vi "radio_get.vi"(0 "VISA in":refnum<visa-resource-name>, 2 "Radio get command":u16(ring) items=["op mode", "frequency", "power", "spread factor", "freq correction", "RX signal bw", "bitrate", "freq deviation", "preamble length", "crc", "bandwidth", "snr"], 5 "error in":errorcluster) -> (14 "VISA out":refnum<visa-resource-name>, 16 "response":string="\r\n", 17 "Num out":u32=57600 max=65535 step=1, 18 "Bool out":bool, 19 "error out":errorcluster)   [LabVIEW 2011]
panel:
  out "read buffer":string
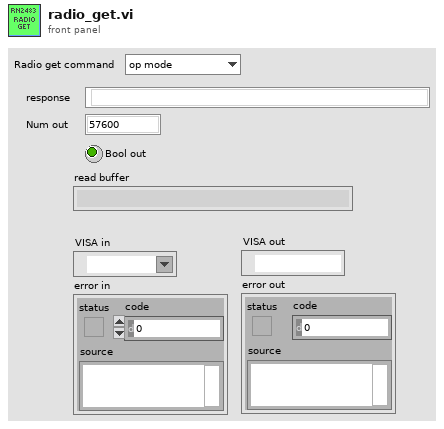
[diagram p1: front panel]
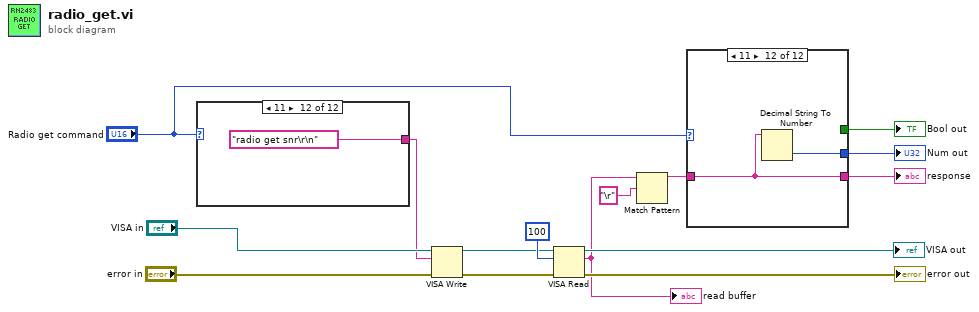
[diagram p0: block diagram]
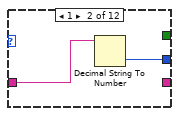
[diagram p3: hidden frame]
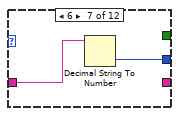
[diagram p8: hidden frame]
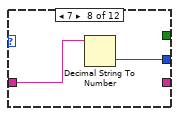
[diagram p9: hidden frame]
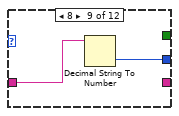
[diagram p10: hidden frame]
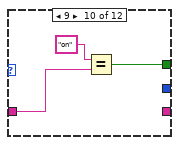
[diagram p11: hidden frame]
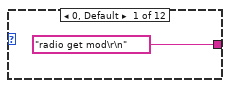
[diagram p13: hidden frame]
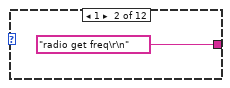
[diagram p14: hidden frame]
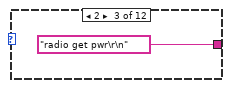
[diagram p15: hidden frame]
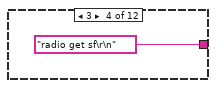
[diagram p16: hidden frame]
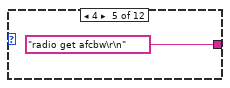
[diagram p17: hidden frame]
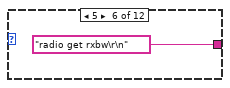
[diagram p18: hidden frame]
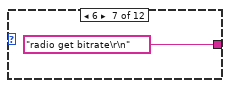
[diagram p19: hidden frame]
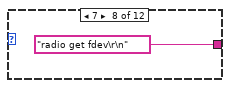
[diagram p20: hidden frame]
diagram:
  n1 = case shown="11" "Radio get command" {
    tunnel: ["radio get mod\r\n" ("string to write") "radio get freq\r\n" ("string to write") "radio get pwr\r\n" ("string to write") "radio get sf\r\n" ("string to write") "radio get afcbw\r\n" ("string to write") "radio get rxbw\r\n" ("string to write") "radio get bitrate\r\n" ("string to write") "radio get fdev\r\n" ("string to write") "radio get prlen\r\n" ("string to write") "radio get crc\r\n" ("string to write") "radio get bw\r\n" ("string to write") "radio get snr\r\n" ("string to write")] -> w8
    frame 0, Default {
    }
    frame 1 {
    }
    frame 2 {
    }
    frame 3 {
    }
    frame 4 {
    }
    frame 5 {
    }
    frame 6 {
    }
    frame 7 {
    }
    frame 8 {
    }
    frame 9 {
    }
    frame 10 {
    }
    frame 11 {
    }
  }
  n2 = VISA Write(VISA resource name="VISA in", write buffer=w8, error in (no error)="error in") -> (VISA resource name out=w10:refnum<visa-resource-name>, error out=w9:errorcluster)  [unwired: 1 out]
  n3 = VISA Read(VISA resource name=w10, byte count=u32 100, error in (no error)=w9) -> (VISA resource name out=→"VISA out":refnum<visa-resource-name>, read buffer=w1:string, error out=→"error out":errorcluster)  [unwired: 1 out]
  "read buffer" <- w1
  n4 = Match Pattern(string=w1, regular expression="\r" ("string to write")) -> (before substring=w2:string)  [unwired: 1 in, 3 out]
  n5 = case shown="11" "Radio get command" {
    tunnel: w2 -> [w28 w30 w31 w32 w33 w34 w36 w38 w40 w42 w44 w46]
    tunnel: [w28 _ w31 w32 w33 w34 _ _ _ _ w44 w46] -> w6
    tunnel: [_ w29 _ _ _ _ w35 w37 w39 _ _ w45] -> w5
    tunnel: [_ _ _ _ _ _ _ _ _ w41 _ _] -> w4
    frame 0, Default {
    }
    frame 1 {
      n6 = Decimal String To Number(string=w30) -> (number=w29:i32)  [unwired: 2 in, 1 out]
    }
    frame 2 {
    }
    frame 3 {
    }
    frame 4 {
    }
    frame 5 {
    }
    frame 6 {
      n7 = Decimal String To Number(string=w36) -> (number=w35:i32)  [unwired: 2 in, 1 out]
    }
    frame 7 {
      n8 = Decimal String To Number(string=w38) -> (number=w37:i32)  [unwired: 2 in, 1 out]
    }
    frame 8 {
      n9 = Decimal String To Number(string=w40) -> (number=w39:i32)  [unwired: 2 in, 1 out]
    }
    frame 9 {
      n10 = Equal?(x="on" ("string to write"), y=w42) -> (x = y?=w41:bool)
    }
    frame 10 {
    }
    frame 11 {
      n11 = Decimal String To Number(string=w46) -> (number=w45:i32)  [unwired: 2 in, 1 out]
    }
  }
  "response" <- w6
  "Num out" <- w5
  "Bool out" <- w4
